vi "OPA.OnShutterStateChanged.vi"(8 "error in (no error)":errorcluster, 10 "Shutter State Changed":T1, 11 "OPA in":refnum<class "OPA.lvclass">) -> (0 "error out":errorcluster, 3 "OPA out":refnum<class "OPA.lvclass">)   [LabVIEW 2017, in "OPA.lvclass"]
uses:
  OPA.lvclass
  Typedefs/PublicEvents--OPA.ShutterStateChanged.ctl
  OPA.lvclass/OPA.ctl
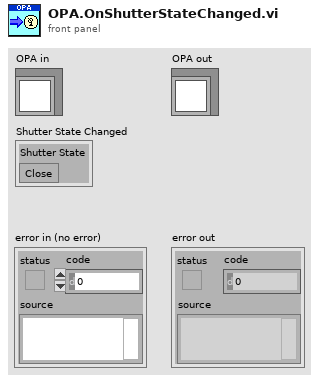
[diagram p1: front panel]
types:
  T1 = typedef "OPA.lvclass/PublicEvents--OPA.ShutterStateChanged.ctl" = cluster{"Shutter State":bool}
  T2 = typedef "OPA.lvclass/PrivateData--Ref.ctl" = refnum<data-value>
  T3 = typedef "OPA.lvclass/PrivateData--Cluster.ctl" = cluster{"Configuration":T4, "Public Events":T5, "Private Events":T6}
  T4 = typedef "OPA.lvclass/Configuration--Cluster.ctl" = cluster{"Serial Number":string}
  T5 = typedef "OPA.lvclass/PublicEvents--Cluster.ctl" = cluster{"WavelengthChanged":refnum<user-event>, "ShutterStateChanged":refnum<user-event>}
  T6 = typedef "OPA.lvclass/PrivateEvents--Cluster.ctl" = cluster{"SetWavelength":refnum<user-event>, "SetShutterState":refnum<user-event>}
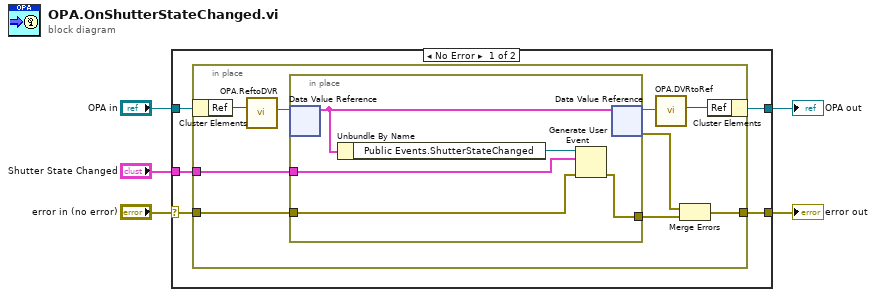
[diagram p0: block diagram]
diagram:
  n1 = case shown="No Error" "error in (no error)" {
    selector: "error in (no error)" -> [w9 w26]
    tunnel: [w8 w26] -> w4
    tunnel: [w7 w25] -> w2
    tunnel: "OPA in" -> [w10 w25]
    tunnel: "Shutter State Changed" -> [w6 _]
    frame No Error {
      n2 = in-place {
        in-place-border: w9 -> [w15]
        in-place-border: [w14] -> w8
        in-place-border: w6 -> [w11]
        n3 = in-place-cluster #1(w10) -> ("Ref"=w19:u32)
        n4 = call "OPA.ReftoDVR.vi"("Ref"=w19) -> ("Ref"=w17:T2)  [unwired: 10 in]
        n5 = in-place {
          in-place-border: w15 -> [w22]
          in-place-border: [w21] -> w12
          in-place-border: w11 -> [w20]
          n6 = in-place-dvr #2(w17) -> (w24:T3)  [unwired: 1 out]
          n7 = Unbundle By Name(w24) -> ("Public Events.ShutterStateChanged"=w23:refnum<user-event>)
          n8 = Generate User Event(user event=w23, event data cluster=w20, error in=w22) -> (error out=w21:errorcluster)  [unwired: 1 in, 1 out]
          n9 = in-place-dvr #2(w24) -> (w16:T2, w13:errorcluster)
        }
        n10 = call "OPA.DVRtoRef.vi"("Ref"=w16) -> ("Ref"=w18:u32)  [unwired: 10 in]
        n11 = Merge Errors(w13, w12) -> (w14:errorcluster)
        n12 = in-place-cluster #1("Ref"=w18) -> (w7:refnum<class "OPA.lvclass">)
      }
    }
    frame Error {
    }
  }
  "error out" <- w4
  "OPA out" <- w2
